vi "BRig_dataRT_stats__FreeReward_c_R.vi"() -> (2 "output_FreeReward_c_R":i32)   [LabVIEW 2014]
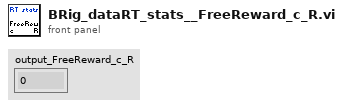
[diagram p1: front panel]
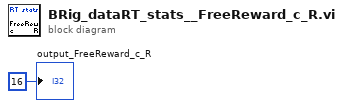
[diagram p0: block diagram]
diagram:
  "output_FreeReward_c_R" <- 16 ("output_iBlock")
